vi "Configure Current Limit.vi"(7 "Channel":i32(ring)=1 items=["Channel 1"=1, "Channel 2"=2, "Channel 3"=3, "Channel 4"=4, "Channel 5"=5, "Channel 6"=6, "Channel 7"=7, "Channel 8"=8, "Channel 8"=9, "Channel 10"=10, "Channel 11"=11, "Channel 12"=12, "Channel 13"=13, "Channel 14"=14, "Channel 15"=15, "Channel 16"=16], 8 "error in":errorcluster, 9 "Limit Type":i32(ring)=1 items=["Low", "High"], 10 "Current(A)":dbl min=0.0, 11 "VISA resource name":refnum<visa-resource-name>) -> (0 "error out":errorcluster, 3 "VISA resource name out":refnum<visa-resource-name>)   [LabVIEW 2020, in "IT-M3400.lvlib"]
doc: "This command is used to set the current limit in voltage priority mode.\n<b>Limit Type</b>\n0:Low\n1:High\n<b>Current(A)</b>\n0-MAX"
uses:
  <instrlib>/IT-M3400/IT-M3400.lvlib
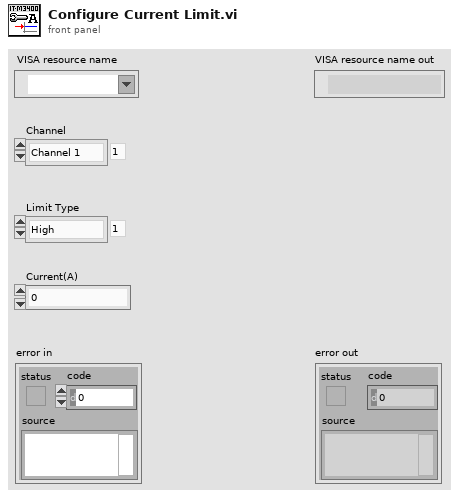
[diagram p1: front panel]
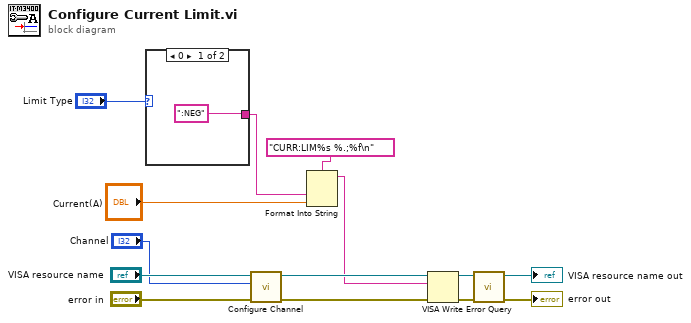
[diagram p0: block diagram]
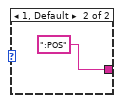
[diagram p2: hidden frame]
diagram:
  n1 = case shown="0" "Limit Type" {
    tunnel: [":NEG" ":POS"] -> w1
    frame 0 {
    }
    frame 1, Default {
    }
  }
  n2 = call <instrlib>:"Configure Channel.vi"("error in"="error in", "Channel"="Channel", "VISA resource name"="VISA resource name") -> ("error out"=w6:errorcluster, "VISA resource name out"=w7:refnum<visa-resource-name>)  [unwired: 7 in]
  n3 = Format Into String(format string="CURR:LIM%s %.;%f\n", w1, "Current(A)") -> (resulting string=w4:string)  [unwired: 2 in, 1 out]
  n4 = VISA Write(VISA resource name=w7, write buffer=w4, error in (no error)=w6) -> (VISA resource name out=w11:refnum<visa-resource-name>, error out=w12:errorcluster)  [unwired: 1 out]
  n5 = call <instrlib>:"Error Query.vi"("error in"=w12, "VISA resource name"=w11) -> ("error out"=→"error out":errorcluster, "VISA resource name out"=→"VISA resource name out":refnum<visa-resource-name>)  [unwired: 6 in, 2 out]
